vi "BufferArray.VI"(9 "Index":i32, 10 "Total amount of Pts":i32, 11 "Input Y-values":dbl[](array[numeric])) -> (3 "Output Array":dbl[](array[numeric]))   [LabVIEW 2014]
panel:
  # "BufferArray.VI"
  # "Inputs"
  # "Outputs"
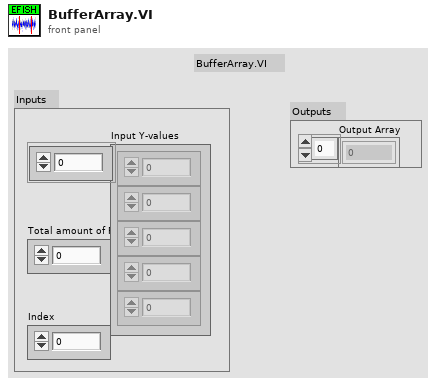
[diagram p1: front panel]
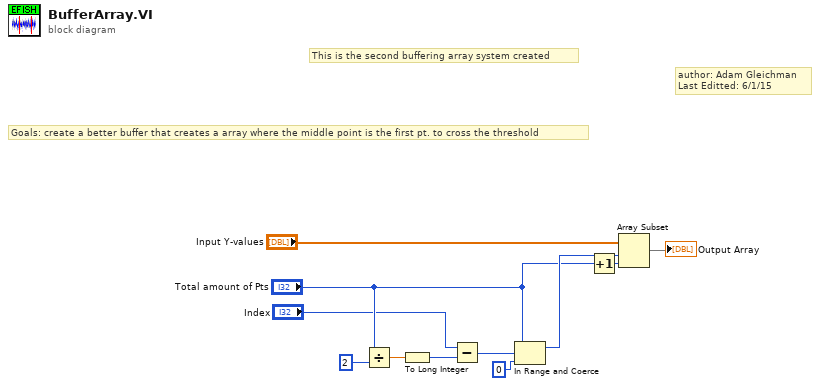
[diagram p0: block diagram]
diagram:
  # "author: Adam Gleichman\nLast Editted: 6/1/15"
  # "This is the second buffering array system created"
  # "Goals: create a better buffer that creates a array where the middle point is the first pt. to cross the threshold"
  n1 = Divide(x="Total amount of Pts", y=2) -> (x/y=w9:dbl)
  n2 = To Long Integer(number=w9) -> (32bit integer=w4:i32)
  n3 = Subtract(x="Index", y=w4) -> (x-y=w2:i32)
  n4 = In Range and Coerce(upper limit="Total amount of Pts", x=w2, lower limit=0) -> (coerced(x)=w7:i32)  [unwired: 1 out]
  n5 = Increment(x="Total amount of Pts") -> (x+1=w1:i32)
  n6 = Array Subset(array="Input Y-values", index=w7, length=w1) -> (→"Output Array":dbl[])
